vi "Teleop.vi"(10 "Match Info":T1={"Autonomous Elapsed Seconds"=0.0, "TeleOp Elapsed Seconds"=0.0, "Disabled Elapsed Seconds"=0.0, "Visited Autonomous"=FALSE, "Visited TeleOp"=FALSE, "Visited Disabled"=FALSE, "Autonomous Settings"={"Autonomous Style"=enum."Independent", "VI Refnum"=refnum}}, 11 "Call Context":T2) -> ()   [LabVIEW 2018]
doc: "This VI is called for each TeleOp packet received from the DS where the robot is not disabled. It is often used to read from the joysticks and update I/O or to update setpoints for timed control loops. It should complete and return within 20 milliseconds or it may miss DS packets."
uses:
  <vilib>/Rock Robotics/WPI/DriverStation/WPI_DriverStationDerivedRobotMode.ctl
  <vilib>/Rock Robotics/WPI/DriverStation/WPI_DriverStationMatch Info.ctl
  <vilib>/Rock Robotics/WPI/Solenoid/WPI_SolenoidValue.ctl
  <vilib>/Rock Robotics/WPI/ThirdParty/Phoenix-LabVIEW/Motor Controller/Controls/CTRE_Phoenix_MotorControl_ControlMode.ctl
  <vilib>/Rock Robotics/WPI/Utilities/WPI_GetSetVariantRefNum.vi
  <vilib>/Rock Robotics/Network Tables/NT Write Boolean Array.vi
  <vilib>/Rock Robotics/Network Tables/NT Write Numeric Array.vi
  <vilib>/Rock Robotics/WPI/Solenoid/WPI_SolenoidSetEnum.vi
  <vilib>/Rock Robotics/Network Tables/NT Write Boolean.vi
  <vilib>/Rock Robotics/WPI/ThirdParty/Phoenix-LabVIEW/Motor Controller/Get/CTRE_Phoenix_MotorController_GetQuadratureData.vi
  <vilib>/Rock Robotics/Network Tables/NT Write Number.vi
  <vilib>/Rock Robotics/Network Tables/NT Read Number.vi
panel:
  out "Angle Ref":dbl
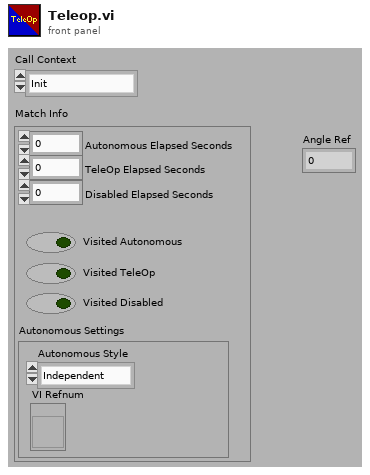
[diagram p1: front panel]
types:
  T1 = typedef "WPI_DriverStationMatch Info.ctl" = cluster{"Autonomous Elapsed Seconds":dbl, "TeleOp Elapsed Seconds":dbl, "Disabled Elapsed Seconds":dbl, "Visited Autonomous":bool, "Visited TeleOp":bool, "Visited Disabled":bool, "Autonomous Settings":cluster{"Autonomous Style":enum16{"Iterative", "Independent"}, "VI Refnum":refnum<vi>}}
  T2 = typedef "WPI_DriverStationDerivedRobotMode.ctl" = enum16{"Init", "Execute", "Stop"}
  T3 = typedef "CTRE_Phoenix_MotorControl_ControlMode.ctl" = u16
  T4 = typedef "WPI_SolenoidValue.ctl" = enum16{"Off", "On", "Forward", "Reverse"}
  T5 = typedef "WPI_JoystickDevRef.ctl" = cluster{"Device":T6}
  T6 = typedef "WPI_JoystickDeviceEnum.ctl" = enum16{"USB 0", "USB 1", "USB 2", "USB 3", "USB 4", "USB 5"}
  T7 = cluster{"Buttons[0]":bool, "Buttons[1]":bool, "Buttons[2]":bool, "Buttons[3]":bool, "Buttons[4]":bool, "Buttons[5]":bool, "Buttons[6]":bool, "Buttons[7]":bool, "Buttons[8]":bool, "Buttons[9]":bool, "Buttons[10]":bool, "Buttons[11]":bool, "Buttons[12]":bool, "Buttons[13]":bool}
  T8 = cluster{"Axes[0]":dbl, "Axes[1]":dbl, "Axes[2]":dbl, "Axes[3]":dbl, "Axes[4]":dbl, "Axes[5]":dbl, "Axes[6]":dbl, "Axes[7]":dbl, "Axes[8]":dbl}
  T9 = typedef "WPI_SolenoidDevRef.ctl" = cluster{"DevStatus":errorcluster, "Pneumatics Control Module":u8, "Forward Solenoid Channel":T10, "Reverse Solenoid Channel":T10}
  T10 = typedef "WPI_SolenoidChannel.ctl" = enum8{"Solenoid 0", "Solenoid 1", "Solenoid 2", "Solenoid 3", "Solenoid 4", "Solenoid 5", "Solenoid 6", "Solenoid 7", "Invalid"}
  T11 = cluster{"Yaw":dbl, "Roll":dbl, "Pitch":dbl, "Heading":dbl, "Fused Heading":dbl}
  T12 = typedef "WPI_MotorControlDeviceRef.ctl" = cluster{"DeviceStatus":errorcluster, "Type":T13, "PWM":cluster{"PWM Channel":T14, "DeadBand":T15}, "CAN":cluster{"Device Number":u8, "SetOutput VI Ref":variant, "GetOutput VI Ref":variant, "Enable VI Ref":variant, "Disable VI Ref":variant, "Data":variant}, "Invert":bool, "DIO PWM":cluster{"PWM \"Enable\" Channel":T14, "DIOChannel":T16, "PWM Rate":dbl}}
  T13 = typedef "WPI_MotorControlType.ctl" = enum16{"PWM", "CAN", "DIO PWM"}
  T14 = typedef "FPGA_DIOPWMChannel.ctl" = enum8{"PWM 0", "PWM 1", "PWM 2", "PWM 3", "PWM 4", "PWM 5", "PWM 6", "PWM 7", "PWM 8", "PWM 9", "PWM MXP 0", "PWM MXP 1", "PWM MXP 2", "PWM MXP 3", "PWM MXP 4", "PWM MXP 5", "PWM MXP 6", "PWM MXP 7", "PWM MXP 8", "PWM MXP 9", "Invalid"}
  T15 = typedef "WPI_PWMDeadband.ctl" = cluster{"Name":string, "maxPositivePwm":i32, "minPositivePwm":i32, "centerPwm":i32, "maxNegativePwm":i32, "minNegativePwm":i32, "angularRange":u16}
  T16 = typedef "FPGA_DIOChannel.ctl" = enum8{"DIO 0", "DIO 1", "DIO 2", "DIO 3", "DIO 4", "DIO 5", "DIO 6", "DIO 7", "DIO 8", "DIO 9", "DIO MXP 0", "DIO MXP 1", "DIO MXP 2", "DIO MXP 3", "DIO MXP 4", "DIO MXP 5", "DIO MXP 6", "DIO MXP 7", "DIO MXP 8", "DIO MXP 9", "DIO MXP 10", "DIO MXP 11", "DIO MXP 12", "DIO MXP 13", "DIO MXP 14", "DIO MXP 15", "SPI Port CS1", "SPI Port CS2", "SPI Port CS3", "SPI Port MISO", "SPI Port MOSI", "Invalid"}
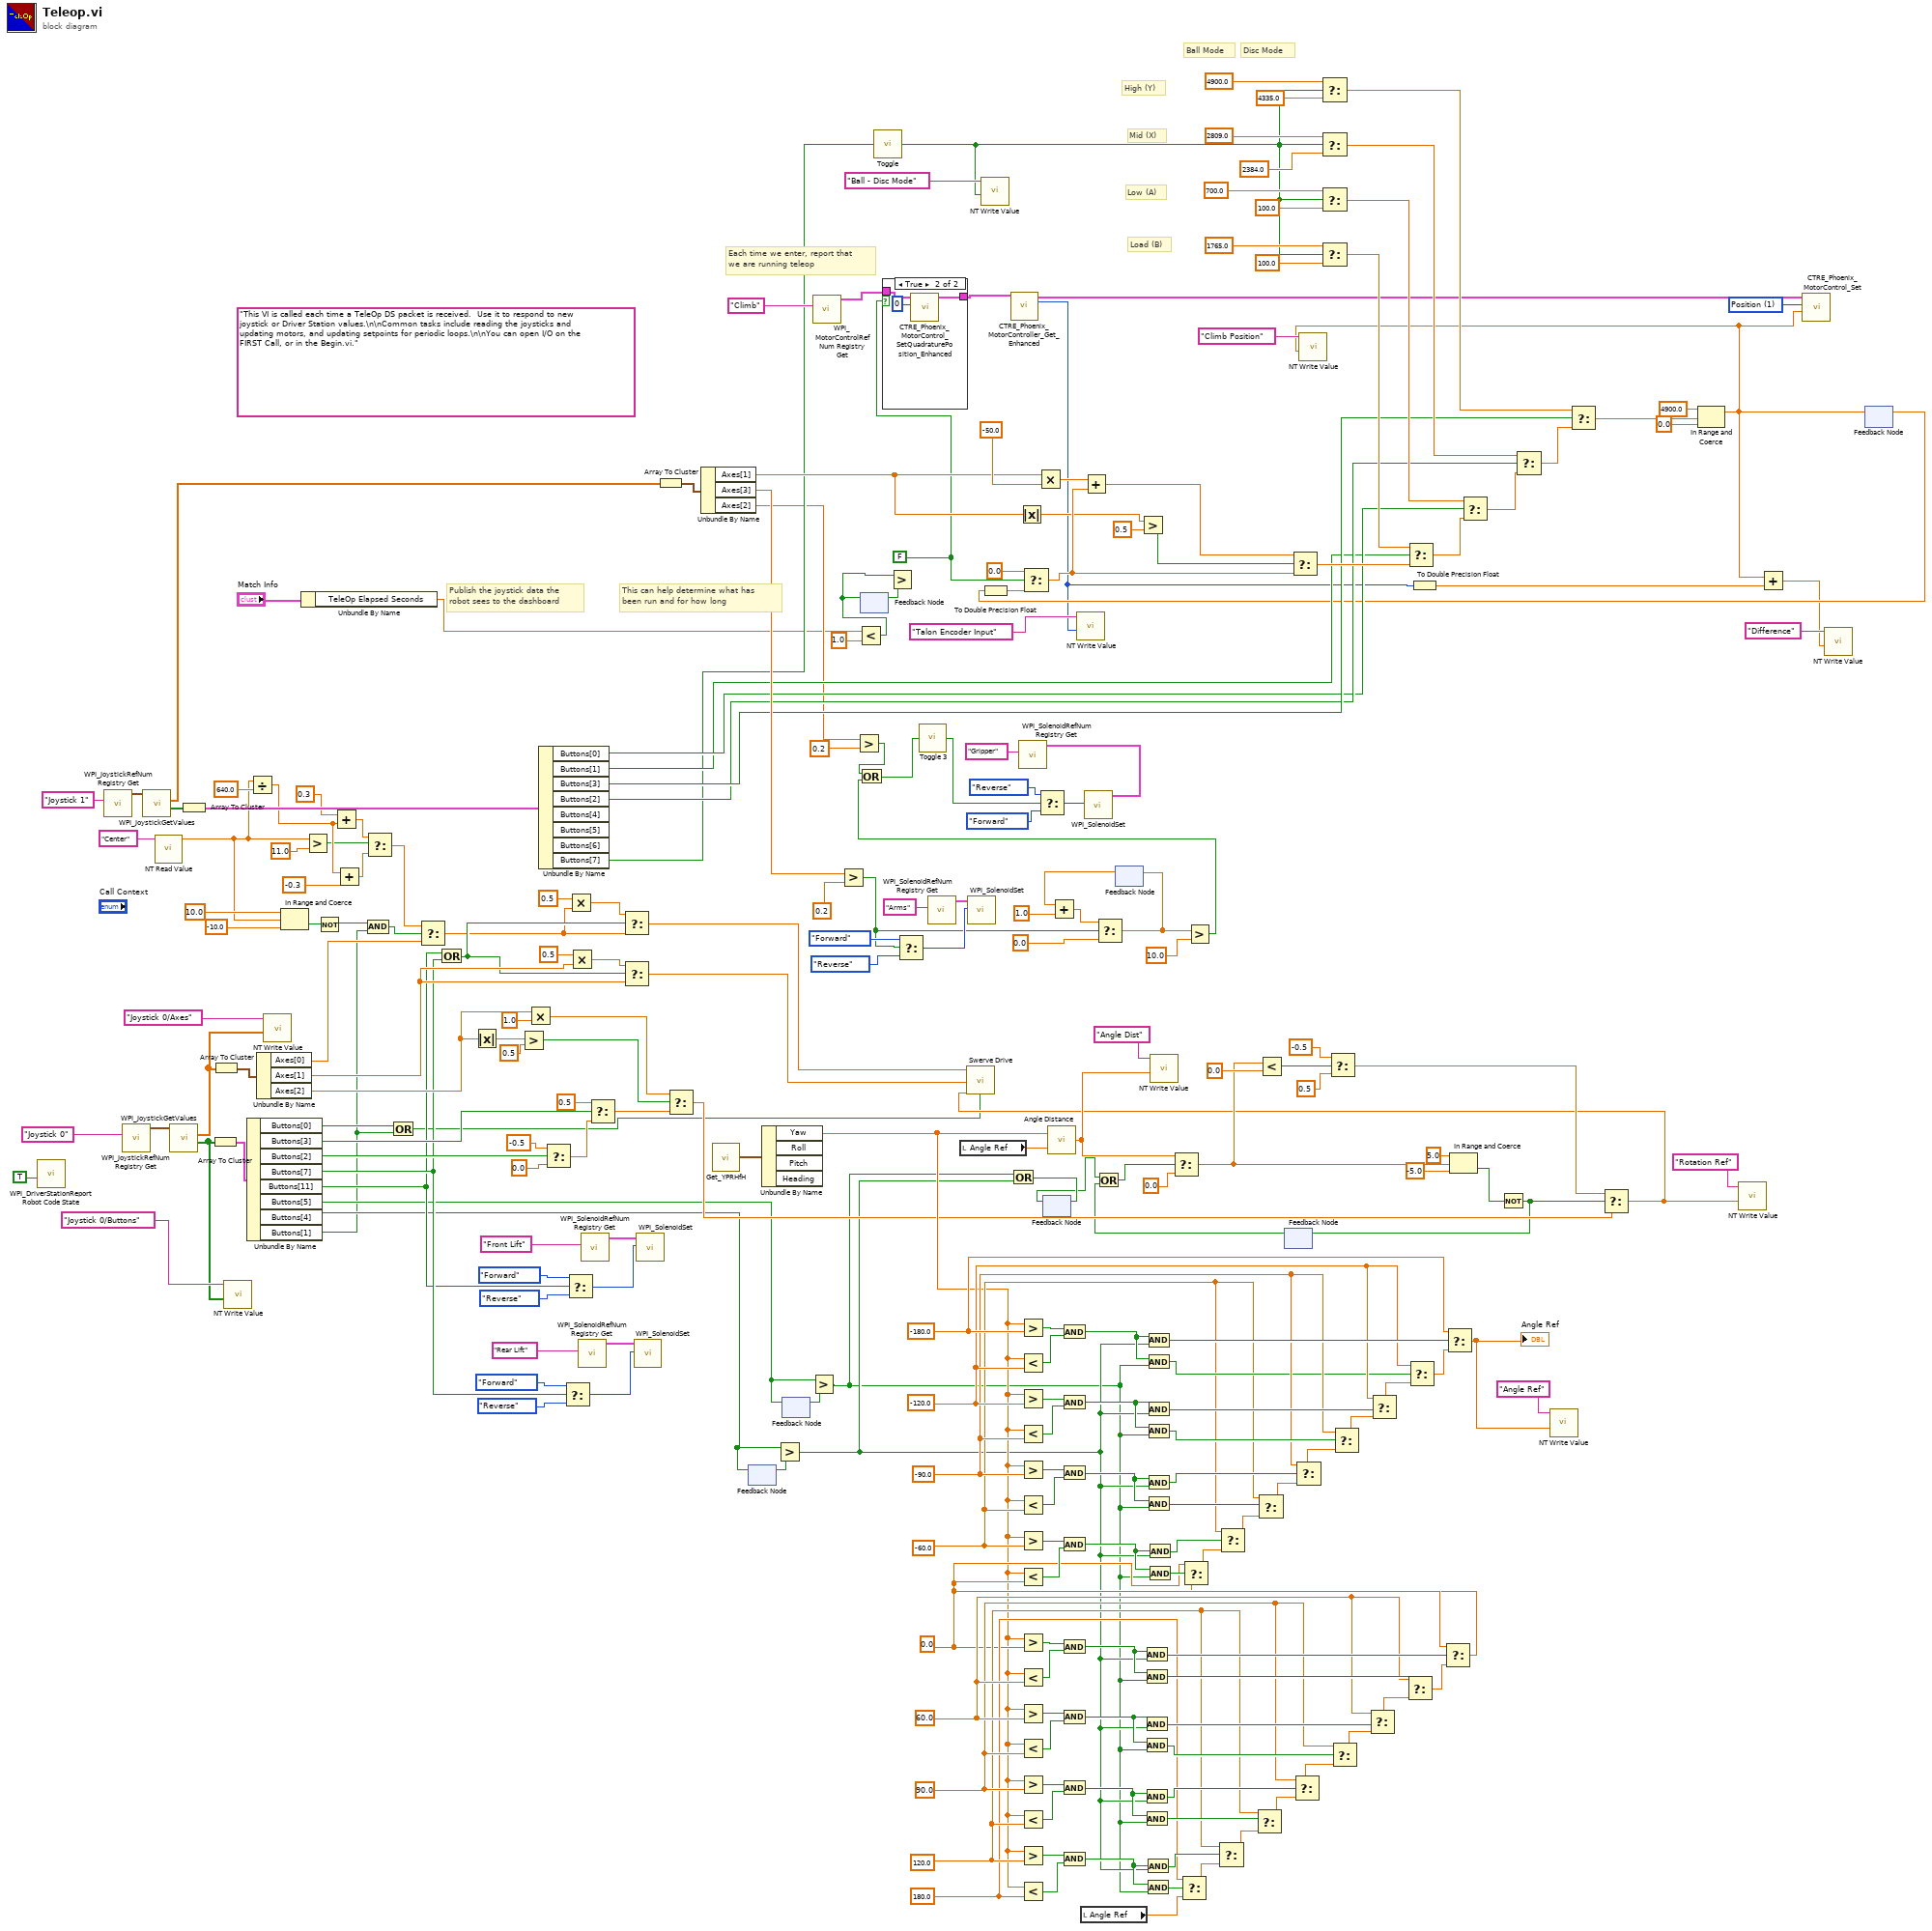
[diagram p0: block diagram]
diagram:
  w32 = FALSE
  w62 = -180.0
  w61 = -120.0
  w60 = -90.0
  w56 = -60.0
  w89 = 180.0
  w90 = 120.0
  w91 = 90.0
  w92 = 60.0
  w59 = 0.0
  w209 = T3 1 items=["PercentOutput"=0, "Position"=1, "Velocity"=2, "Current"=3, "Follower"=5, "MotionProfile"=6, "MotionMagic"=7, "MotionProfileArc"=10, "Disabled"=15] ("Control Mode")
  (unwired) "This VI is called each time a TeleOp DS packet is received.  Use it to respond to new joystick or Driver Station values.\n\nCommon tasks include reading the joysticks and updating motors, and updating setpoints for periodic loops.\n\nYou can open I/O on the FIRST Call, or in the Begin.vi."
  # "High (Y)"
  # "Mid (X)"
  # "Low (A)"
  # "Load (B)"
  # "Disc Mode"
  # "Ball Mode"
  # "Publish the joystick data the\nrobot sees to the dashboard"
  # "Each time we enter, report that\nwe are running teleop"
  # "This can help determine what has\nbeen run and for how long"
  n1 = call <vilib>:"WPI_DriverStationReport Robot Code State.vi"("TeleOp"=TRUE ("Autonomous")) -> ()  [unwired: 10 in, 1 out]
  n2 = call <vilib>:"WPI_JoystickRefNum Registry Get.vi"("refnum name"="Joystick 1") -> ("JoystickDevRef"=w216:T5)  [unwired: 1 in, 9 out]
  n3 = call <vilib>:"WPI_JoystickRefNum Registry Get.vi"("refnum name"="Joystick 0") -> ("JoystickDevRef"=w243:T5)  [unwired: 1 in, 9 out]
  n4 = call <vilib>:"WPI_JoystickGetValues.vi"("JoystickDevRef"=w216) -> ("Buttons"=w214:bool[], "Axes"=w210:dbl[])  [unwired: 6 in, 3 out]
  n5 = call-poly <vilib>:"NT Read Value.vi"("Name"="Center" ("refnum name")) -> ("Numeric"=w3:dbl)  [unwired: 9 in, 1 out]
  n6 = call <vilib>:"WPI_JoystickGetValues.vi"("JoystickDevRef"=w243) -> ("Buttons"=w237:bool[], "Axes"=w239:dbl[])  [unwired: 6 in, 3 out]
  n7 = Array To Cluster(array=w214) -> (cluster=w213:T7)
  n8 = Array To Cluster(array=w237) -> (cluster=w236:T7)
  n9 = Array To Cluster(array=w239) -> (cluster=w238:T8)
  n10 = call-poly <vilib>:"NT Write Value.vi"("Boolean Array"=w237, "Name"="Joystick 0/Buttons") -> ()  [unwired: 9 in, 1 out]
  n11 = Unbundle By Name(w236) -> ("Buttons[0]"=w17:bool, "Buttons[3]"=w131:bool, "Buttons[2]"=w132:bool, "Buttons[7]"=w49:bool, "Buttons[11]"=w48:bool, "Buttons[5]"=w31:bool, "Buttons[4]"=w29:bool, "Buttons[1]"=w13:bool)
  n12 = Divide(x=w3, y=640.0) -> (x/y=w2:dbl)
  n13 = Unbundle By Name(w238) -> ("Axes[0]"=w21:dbl, "Axes[1]"=w51:dbl, "Axes[2]"=w138:dbl)
  n14 = call-poly <vilib>:"NT Write Value.vi"("Numeric Array"=w239, "Name"="Joystick 0/Axes") -> ()  [unwired: 9 in, 1 out]
  n15 = In Range and Coerce(upper limit=10.0, x=w3, lower limit=-10.0) -> (In Range?=w11:bool)  [unwired: 1 out]
  n16 = Unbundle By Name("Match Info") -> ("TeleOp Elapsed Seconds"=w150:dbl)
  n17 = Greater?(x=w3, y=11.0) -> (0:w1:bool)
  n18 = Not(x=w11) -> (.not. x?=w12:bool)
  n19 = Add(x=0.3 ("t"), y=w2) -> (x+y=w7:dbl)
  n20 = Add(x=w2, y=-0.3 ("f")) -> (x+y=w8:dbl)
  n21 = And(x=w12, y=w13) -> (x .and. y?=w10:bool)
  n22 = Select(t=w7, s=w1, f=w8) -> (s? t:f=w19:dbl)
  n23 = Or(x=w17, y=w13) -> (x .or. y?=w16:bool)
  n24 = Select(t=w19, s=w10, f=w21) -> (s? t:f=w20:dbl)
  n25 = Or(x=w48, y=w49) -> (x .or. y?=w47:bool)
  n26 = Absolute Value(x=w138) -> (abs(x)=w141:dbl)
  n27 = Greater?(x=w141, y=0.5) -> (0:w130:bool)
  n28 = Multiply(x=w138, y=1.0) -> (x*y=w139:dbl)
  n29 = Unbundle By Name(w213) -> ("Buttons[0]"=w175:bool, "Buttons[1]"=w174:bool, "Buttons[3]"=w177:bool, "Buttons[2]"=w176:bool, "Buttons[7]"=w172:bool)  [unwired: 3 out]
  n30 = Select(t=-0.5, s=w132, f=0.0) -> (s? t:f=w136:dbl)
  n31 = Select(t=WPI_SolenoidValue."Forward" ("Value"), s=w49, f=WPI_SolenoidValue."Reverse") -> (s? t:f=w219:T4)
  n32 = Select(t=WPI_SolenoidValue."Forward" ("Value"), s=w48, f=WPI_SolenoidValue."Reverse") -> (s? t:f=w218:T4)
  n33 = Multiply(x=0.5, y=w20) -> (x*y=w50:dbl)
  n34 = Multiply(x=0.5, y=w51) -> (x*y=w52:dbl)
  n35 = call <vilib>:"WPI_SolenoidRefNum Registry Get.vi"("refnum name"="Rear Lift") -> ("SolenoidDevRef"=w229:T9)  [unwired: 9 in, 1 out]
  n36 = call <vilib>:"WPI_SolenoidRefNum Registry Get.vi"("refnum name"="Front Lift") -> ("SolenoidDevRef"=w230:T9)  [unwired: 9 in, 1 out]
  n37 = Select(t=0.5, s=w131, f=w136) -> (s? t:f=w129:dbl)
  n38 = Select(t=w50, s=w47, f=w20) -> (s? t:f=w45:dbl)
  n39 = Select(t=w52, s=w47, f=w51) -> (s? t:f=w46:dbl)
  n40 = call-poly <vilib>:"WPI_SolenoidSet.vi"("Value"=w219, "SolenoidDevRef"=w229) -> ()  [unwired: 8 in, 2 out]
  n41 = call-poly <vilib>:"WPI_SolenoidSet.vi"("Value"=w218, "SolenoidDevRef"=w230) -> ()  [unwired: 8 in, 2 out]
  n42 = Array To Cluster(array=w210) -> (cluster=w211:T8)
  n43 = Select(t=w139, s=w130, f=w129) -> (s? t:f=w40:dbl)
  n44 = Unbundle By Name(w211) -> ("Axes[1]"=w197:dbl, "Axes[3]"=w204:dbl, "Axes[2]"=w170:dbl)
  n45 = call <vilib>:"Get_YPRHfH.vi"() -> ("YRPHfH"=w128:T11)  [unwired: 11 in]
  n46 = feedback #1() -> (w42:bool)  [unwired: 1 in]
  n47 = feedback-in #1(w29) -> ()
  n48 = Unbundle By Name(w128) -> ("Yaw"=w55:dbl)  [unwired: 3 out]
  n49 = Greater?(x=w29, y=w42) -> (0:w23:bool)
  n50 = feedback #2() -> (w43:bool)  [unwired: 1 in]
  n51 = feedback-in #2(w31) -> ()
  n52 = Greater?(x=w31, y=w43) -> (0:w22:bool)
  n53 = call <vilib>:"WPI_MotorControlRefNum Registry Get.vi"("refnum name"="Climb") -> ("MotorControlDevRef"=w154:T12)  [unwired: 9 in, 1 out]
  n54 = Greater?(x=w204, y=0.2) -> (0:w167:bool)
  n55 = Greater?(x=w170, y=0.2) -> (0:w160:bool)
  n56 = Less?(x=w150, y=1.0) -> (x < y?=w151:bool)
  n57 = feedback-in #3(w151) -> ()
  n58 = feedback #3() -> (w152:bool)  [unwired: 1 in]
  n59 = call "Toggle.vi"("Input"=w172) -> ("Output"=w156:bool)
  n60 = case shown="True" w32 {
    tunnel: w154 -> [w246 w249]
    tunnel: [w246 w248] -> w153
    frame False {
    }
    frame True {
      n61 = call <vilib>:"CTRE_Phoenix_MotorControl_SetQuadraturePosition_Enhanced.vi"("New Position"=0, "PhoenixMotorControlDevRef"=w249) -> ("PhoenixMotorControlDevRef"=w248:T12)  [unwired: 8 in, 1 out]
    }
  }
  n62 = Greater?(x=w151, y=w152) -> ()  [unwired: 1 out]
  n63 = Select(t=WPI_SolenoidValue."Forward" ("Value"), s=w167, f=WPI_SolenoidValue."Reverse") -> (s? t:f=w232:T4)
  n64 = call <vilib>:"WPI_SolenoidRefNum Registry Get.vi"("refnum name"="Arms") -> ("SolenoidDevRef"=w234:T9)  [unwired: 9 in, 1 out]
  n65 = local read "Angle Ref"() -> (w44:dbl)
  n66 = call-poly <vilib>:"WPI_SolenoidSet.vi"("Value"=w232, "SolenoidDevRef"=w234) -> ()  [unwired: 8 in, 2 out]
  n67 = call-poly <vilib>:"NT Write Value.vi"("Boolean"=w156, "Name"="Ball - Disc Mode") -> ()  [unwired: 9 in, 1 out]
  n68 = Or(x=w22, y=w23) -> (x .or. y?=w25:bool)
  n69 = call-poly <vilib>:"CTRE_Phoenix_MotorController_Get_Enhanced.vi"("PhoenixMotorControlDevRef"=w153) -> ("PhoenixMotorControlDevRef"=w158:T12, "Quadrature Position"=w145:i32)  [unwired: 11 in, 2 out]
  n70 = Absolute Value(x=w197) -> (abs(x)=w196:dbl)
  n71 = call <vilib>:"WPI_SolenoidRefNum Registry Get.vi"("refnum name"="Gripper") -> ("SolenoidDevRef"=w231:T9)  [unwired: 9 in, 1 out]
  n72 = Greater?(x=w55, y=w62) -> (0:w88:bool)
  n73 = Less?(x=w55, y=w61) -> (x < y?=w87:bool)
  n74 = Greater?(x=w55, y=w61) -> (0:w83:bool)
  n75 = Less?(x=w55, y=w60) -> (x < y?=w82:bool)
  n76 = Greater?(x=w55, y=w60) -> (0:w81:bool)
  n77 = Less?(x=w55, y=w56) -> (x < y?=w80:bool)
  n78 = Greater?(x=w55, y=w56) -> (0:w79:bool)
  n79 = Less?(x=w55, y=w59) -> (x < y?=w78:bool)
  n80 = Greater?(x=w55, y=w59) -> (0:w119:bool)
  n81 = Less?(x=w55, y=w92) -> (x < y?=w118:bool)
  n82 = Greater?(x=w55, y=w92) -> (0:w113:bool)
  n83 = Less?(x=w55, y=w91) -> (x < y?=w112:bool)
  n84 = Greater?(x=w55, y=w91) -> (0:w111:bool)
  n85 = Less?(x=w55, y=w90) -> (x < y?=w110:bool)
  n86 = Greater?(x=w55, y=w90) -> (0:w109:bool)
  n87 = Less?(x=w55, y=w89) -> (x < y?=w108:bool)
  n88 = Multiply(x=w197, y=-50.0) -> (x*y=w202:dbl)
  n89 = feedback-in #4(w25) -> ()
  n90 = feedback #4() -> (w24:bool)  [unwired: 1 in]
  n91 = call "Angle Distance.vi"("target angle"=w44, "current angle"=w55) -> ("distance"=w35:dbl)
  n92 = And(x=w88, y=w87) -> (x .and. y?=w86:bool)
  n93 = And(x=w83, y=w82) -> (x .and. y?=w77:bool)
  n94 = And(x=w81, y=w80) -> (x .and. y?=w76:bool)
  n95 = And(x=w79, y=w78) -> (x .and. y?=w75:bool)
  n96 = And(x=w119, y=w118) -> (x .and. y?=w117:bool)
  n97 = And(x=w113, y=w112) -> (x .and. y?=w107:bool)
  n98 = And(x=w111, y=w110) -> (x .and. y?=w106:bool)
  n99 = And(x=w109, y=w108) -> (x .and. y?=w105:bool)
  n100 = call-poly <vilib>:"NT Write Value.vi"("Numeric"=w145, "Name"="Talon Encoder Input") -> ()  [unwired: 9 in, 1 out]
  n101 = local read "Angle Ref"() -> (w30:dbl)
  n102 = feedback #5() -> (w163:dbl)  [unwired: 1 in]
  n103 = Add(x=w163, y=1.0) -> (x+y=w165:dbl)
  n104 = Select(t=w165, s=w167, f=0.0) -> (s? t:f=w162:dbl)
  n105 = feedback-in #5(w162) -> ()
  n106 = Greater?(x=w196, y=0.5) -> (0:w195:bool)
  n107 = And(x=w117, y=w23) -> (x .and. y?=w116:bool)
  n108 = And(x=w117, y=w22) -> (x .and. y?=w115:bool)
  n109 = And(x=w107, y=w23) -> (x .and. y?=w98:bool)
  n110 = And(x=w107, y=w22) -> (x .and. y?=w97:bool)
  n111 = And(x=w106, y=w23) -> (x .and. y?=w96:bool)
  n112 = And(x=w106, y=w22) -> (x .and. y?=w95:bool)
  n113 = And(x=w105, y=w23) -> (x .and. y?=w94:bool)
  n114 = And(x=w105, y=w22) -> (x .and. y?=w93:bool)
  n115 = And(x=w86, y=w23) -> (x .and. y?=w85:bool)
  n116 = And(x=w86, y=w22) -> (x .and. y?=w57:bool)
  n117 = And(x=w77, y=w23) -> (x .and. y?=w68:bool)
  n118 = And(x=w77, y=w22) -> (x .and. y?=w67:bool)
  n119 = And(x=w76, y=w23) -> (x .and. y?=w66:bool)
  n120 = And(x=w76, y=w22) -> (x .and. y?=w65:bool)
  n121 = And(x=w75, y=w23) -> (x .and. y?=w64:bool)
  n122 = And(x=w75, y=w22) -> (x .and. y?=w63:bool)
  n123 = call-poly <vilib>:"NT Write Value.vi"("Numeric"=w35, "Name"="Angle Dist") -> ()  [unwired: 9 in, 1 out]
  n124 = Select(t=w89, s=w93, f=w30) -> (s? t:f=w99:dbl)
  n125 = Greater?(x=w162, y=10.0) -> (0:w159:bool)
  n126 = Or(x=w160, y=w159) -> (x .or. y?=w157:bool)
  n127 = call "Toggle 3.vi"("Input"=w157) -> ("Output"=w168:bool)
  n128 = Select(t=WPI_SolenoidValue."Reverse" ("Value"), s=w168, f=WPI_SolenoidValue."Forward") -> (s? t:f=w217:T4)
  n129 = call-poly <vilib>:"WPI_SolenoidSet.vi"("Value"=w217, "SolenoidDevRef"=w231) -> ()  [unwired: 8 in, 2 out]
  n130 = Select(t=w90, s=w94, f=w99) -> (s? t:f=w100:dbl)
  n131 = Select(t=w90, s=w95, f=w100) -> (s? t:f=w101:dbl)
  n132 = feedback #6() -> (w27:bool)  [unwired: 1 in]
  n133 = Or(x=w24, y=w27) -> (x .or. y?=w26:bool)
  n134 = Select(t=w35, s=w26, f=0.0) -> (s? t:f=w123:dbl)
  n135 = Less?(x=w123, y=0.0) -> (x < y?=w122:bool)
  n136 = Select(t=w91, s=w96, f=w101) -> (s? t:f=w102:dbl)
  n137 = Select(t=4900.0, s=w156, f=4335.0) -> (s? t:f=w188:dbl)
  n138 = Select(t=2809.0, s=w156, f=2384.0) -> (s? t:f=w189:dbl)
  n139 = Select(t=700.0, s=w156, f=100.0) -> (s? t:f=w190:dbl)
  n140 = Select(t=1765.0, s=w156, f=100.0) -> (s? t:f=w191:dbl)
  n141 = Select(t=-0.5, s=w122, f=0.5) -> (s? t:f=w39:dbl)
  n142 = Select(t=w91, s=w97, f=w102) -> (s? t:f=w103:dbl)
  n143 = Select(t=w92, s=w98, f=w103) -> (s? t:f=w104:dbl)
  n144 = Select(t=w92, s=w115, f=w104) -> (s? t:f=w114:dbl)
  n145 = To Double Precision Float(number=w145) -> (double precision float=w144:dbl)
  n146 = Select(t=w59, s=w116, f=w114) -> (s? t:f=w58:dbl)
  n147 = Select(t=w59, s=w63, f=w58) -> (s? t:f=w69:dbl)
  n148 = Select(t=w56, s=w64, f=w69) -> (s? t:f=w70:dbl)
  n149 = Select(t=w56, s=w65, f=w70) -> (s? t:f=w71:dbl)
  n150 = Select(t=w60, s=w66, f=w71) -> (s? t:f=w72:dbl)
  n151 = Select(t=w60, s=w67, f=w72) -> (s? t:f=w73:dbl)
  n152 = Select(t=w61, s=w68, f=w73) -> (s? t:f=w74:dbl)
  n153 = Select(t=w61, s=w57, f=w74) -> (s? t:f=w84:dbl)
  n154 = Select(t=w62, s=w85, f=w84) -> (s? t:f=w37:dbl)
  "Angle Ref" <- w37
  n155 = In Range and Coerce(upper limit=5.0, x=w123, lower limit=-5.0) -> (In Range?=w41:bool)  [unwired: 1 out]
  n156 = Not(x=w41) -> (.not. x?=w28:bool)
  n157 = feedback-in #6(w28) -> ()
  n158 = call-poly <vilib>:"NT Write Value.vi"("Numeric"=w37, "Name"="Angle Ref") -> ()  [unwired: 9 in, 1 out]
  n159 = Select(t=w39, s=w28, f=w40) -> (s? t:f=w33:dbl)
  n160 = call "Swerve Drive.vi"("X"=w45, "Y"=w46, "Z"=w33, "Robot-Centric"=w16) -> ()  [unwired: 12 in]
  n161 = call-poly <vilib>:"NT Write Value.vi"("Numeric"=w33, "Name"="Rotation Ref") -> ()  [unwired: 9 in, 1 out]
  n162 = feedback #7() -> (w147:dbl)  [unwired: 1 in]
  n163 = To Double Precision Float(number=w147) -> (double precision float=w148:dbl)
  n164 = Select(t=0.0, s=w32, f=w148) -> (s? t:f=w198:dbl)
  n165 = Add(x=w202, y=w198) -> (x+y=w199:dbl)
  n166 = Select(t=w199, s=w195, f=w198) -> (s? t:f=w187:dbl)
  n167 = Select(t=w191, s=w174, f=w187) -> (s? t:f=w194:dbl)
  n168 = Select(t=w190, s=w175, f=w194) -> (s? t:f=w193:dbl)
  n169 = Select(t=w189, s=w176, f=w193) -> (s? t:f=w192:dbl)
  n170 = Select(t=w188, s=w177, f=w192) -> (s? t:f=w186:dbl)
  n171 = In Range and Coerce(upper limit=4900.0, x=w186, lower limit=0.0) -> (coerced(x)=w146:dbl)  [unwired: 1 out]
  n172 = call-poly <vilib>:"NT Write Value.vi"("Numeric"=w146, "Name"="Climb Position") -> ()  [unwired: 9 in, 1 out]
  n173 = Add(x=w146, y=w144) -> (x+y=w142:dbl)
  n174 = call <vilib>:"CTRE_Phoenix_MotorControl_Set.vi"("Output"=w146, "Control Mode"=w209, "PhoenixMotorControlDevRef"=w158) -> ()  [unwired: 7 in, 2 out]
  n175 = call-poly <vilib>:"NT Write Value.vi"("Numeric"=w142, "Name"="Difference") -> ()  [unwired: 9 in, 1 out]
  n176 = feedback-in #7(w146) -> ()
